vi "Interpolate 1 Table BY DP.vi"(1 "First Known Value":dbl, 7 "Psych Table, 1 Press., 1 DP":dbl[][](array[numeric])=[[1000.0, 14.17265118, 0.0, -0.621764104, 80.0, 0.000650233, 4.551631867, 12.02925562, 0.689897344, -4.171510822], [1000.0, 14.17265118, 5.0, 4.228401567, 80.0, 0.000842818, 5.899726242, 12.16386356, 2.096100991, 0.713093012], [1000.0, 14.17265118, 10.0, 9.054425448, 80.0, 0.001086491, 7.605438605, 12.29956097, 3.557591215, 5.60922632], [1000.0, 14.17265118, 15.0, 13.85608869, 80.0, 0.00139325, 9.752748458, 12.43661941, 5.08751706, 10.51277979], [1000.0, 14.17265118, 20.0, 18.63419614, 80.0, 0.001777556, 12.44289539, 12.57537024, 6.701772131, 15.41996209], [1000.0, 14.17265118, 25.0, 23.39061149, 80.0, 0.002256784, 15.79748474, 12.71621624, 8.419497627, 20.32727624], [1000.0, 14.17265118, 30.0, 28.12820033, 80.0, 0.00285173, 19.96211141, 12.85964533, 10.26367079, 25.2314979], [1000.0, 14.17265118, 35.0, 32.7497224, 80.0, 0.003529771, 24.70839817, 13.00505214, 12.19993985, 29.38106424], [1000.0, 14.17265118, 40.0, 37.4647332, 80.0, 0.004302885, 30.12019294, 13.15274062, 14.24177991, 34.32158079], [1000.0, 14.17265118, 45.0, 42.16998509, 80.0, 0.00522362, 36.56533789, 13.30388537, 16.44662842, 39.23751693], [1000.0, 14.17265118, 50.0, 46.86847898, 80.0, 0.006316212, 44.21348175, 13.45909864, 18.84172049, 44.13372432], [1000.0, 14.17265118, 55.0, 51.56310352, 80.0, 0.007608335, 53.25834337, 13.61908743, 21.45823872, 49.01435336], [1000.0, 14.17265118, 60.0, 56.25650983, 80.0, 0.009131564, 63.92094782, 13.78466719, 24.33185424, 53.88293123], [1000.0, 14.17265118, 65.0, 60.95101979, 80.0, 0.010921915, 76.45340424, 13.95677788, 27.50335816, 58.74243194], [1000.0, 14.17265118, 70.0, 65.64857135, 80.0, 0.01302048, 91.14335768, 14.13650272, 31.01940544, 63.59533911], [1000.0, 14.17265118, 75.0, 70.35069813, 80.0, 0.015474184, 108.3192857, 14.32509057, 34.93339919, 68.4437021], [1000.0, 14.17265118, 80.0, 75.05853782, 80.0, 0.018336694, 128.3568607, 14.52398268, 39.30655212, 73.28918652], [1000.0, 14.17265118, 85.0, 79.77286177, 80.0, 0.021669524, 151.6866657, 14.73484497, 44.20917244, 78.13311928], [1000.0, 14.17265118, 90.0, 84.49411846, 80.0, 0.025543377, 178.8036408, 14.9596075, 49.72223662, 82.97652911], [1000.0, 14.17265118, 95.0, 89.22248393, 80.0, 0.030039822, 210.2787556, 15.20051297, 55.93933108, 87.82018277], [1000.0, 14.17265118, 100.0, 93.95791383, 80.0, 0.035253367, 246.7735709, 15.46017708, 62.96907218, 92.66461748], [1000.0, 14.17265118, 105.0, 98.70019305, 80.0, 0.041294082, 289.0585757, 15.74166432, 70.93815137, 97.51017001], [1000.0, 14.17265118, 110.0, 103.4489805, 80.0, 0.048290929, 338.0365051, 16.04858402, 79.99520498, 102.3570026], [1000.0, 14.17265118, 115.0, 108.2038476, 80.0, 0.056396043, 394.7722978, 16.38521366, 90.31578307, 107.2051264], [1000.0, 14.17265118, 120.0, 112.9643104, 80.0, 0.065790285, 460.5319982, 16.75665854, 102.1087993, 112.0544218]], 12 "First Known Index":u16(ring) items=["DB", "WB", "RH", "HR", "Gr", "Vol", "h", "Dp"]) -> (8 "Output Array":dbl[](array[numeric]))   [LabVIEW 2020]
uses:
  <vilib>/gmath/NI_Gmath.lvlib
panel:
  out "deleted portion 1":i32
  out "Out 6":dbl
  out "Property 6":u16(ring) items=["DB", "WB", "RH", "HR", "Gr", "Vol", "h", "Dp"]
  out "deleted portion 3":i32
  out "array 3 w/ subset deleted":i32[](array[numeric])
  out "Property 5":u16(ring) items=["DB", "WB", "RH", "HR", "Gr", "Vol", "h", "Dp"]
  out "Property 4":u16(ring) items=["DB", "WB", "RH", "HR", "Gr", "Vol", "h", "Dp"]
  out "Property 3":u16(ring) items=["DB", "WB", "RH", "HR", "Gr", "Vol", "h", "Dp"]
  out "Property 2":u16(ring) items=["DB", "WB", "RH", "HR", "Gr", "Vol", "h", "Dp"]
  out "Property 1":u16(ring) items=["DB", "WB", "RH", "HR", "Gr", "Vol", "h", "Dp"]
  out "Table without elev and P":dbl[][](array[numeric])
  out "array 1 w/ subset deleted":i32[](array[numeric])
  out "Out 1":dbl
  out "Out 5":dbl
  out "Out 4":dbl
  out "Out 2":dbl
  out "Out 3":dbl
  # "will not work if DP is first known value"
  # "DB"
  # "WB"
  # "RH"
  # "HR"
  # "Gr"
  # "v"
  # "h"
  # "DP"
  # "0"
  # "1"
  # "2"
  # "3"
  # "4"
  # "5"
  # "6"
  # "7"
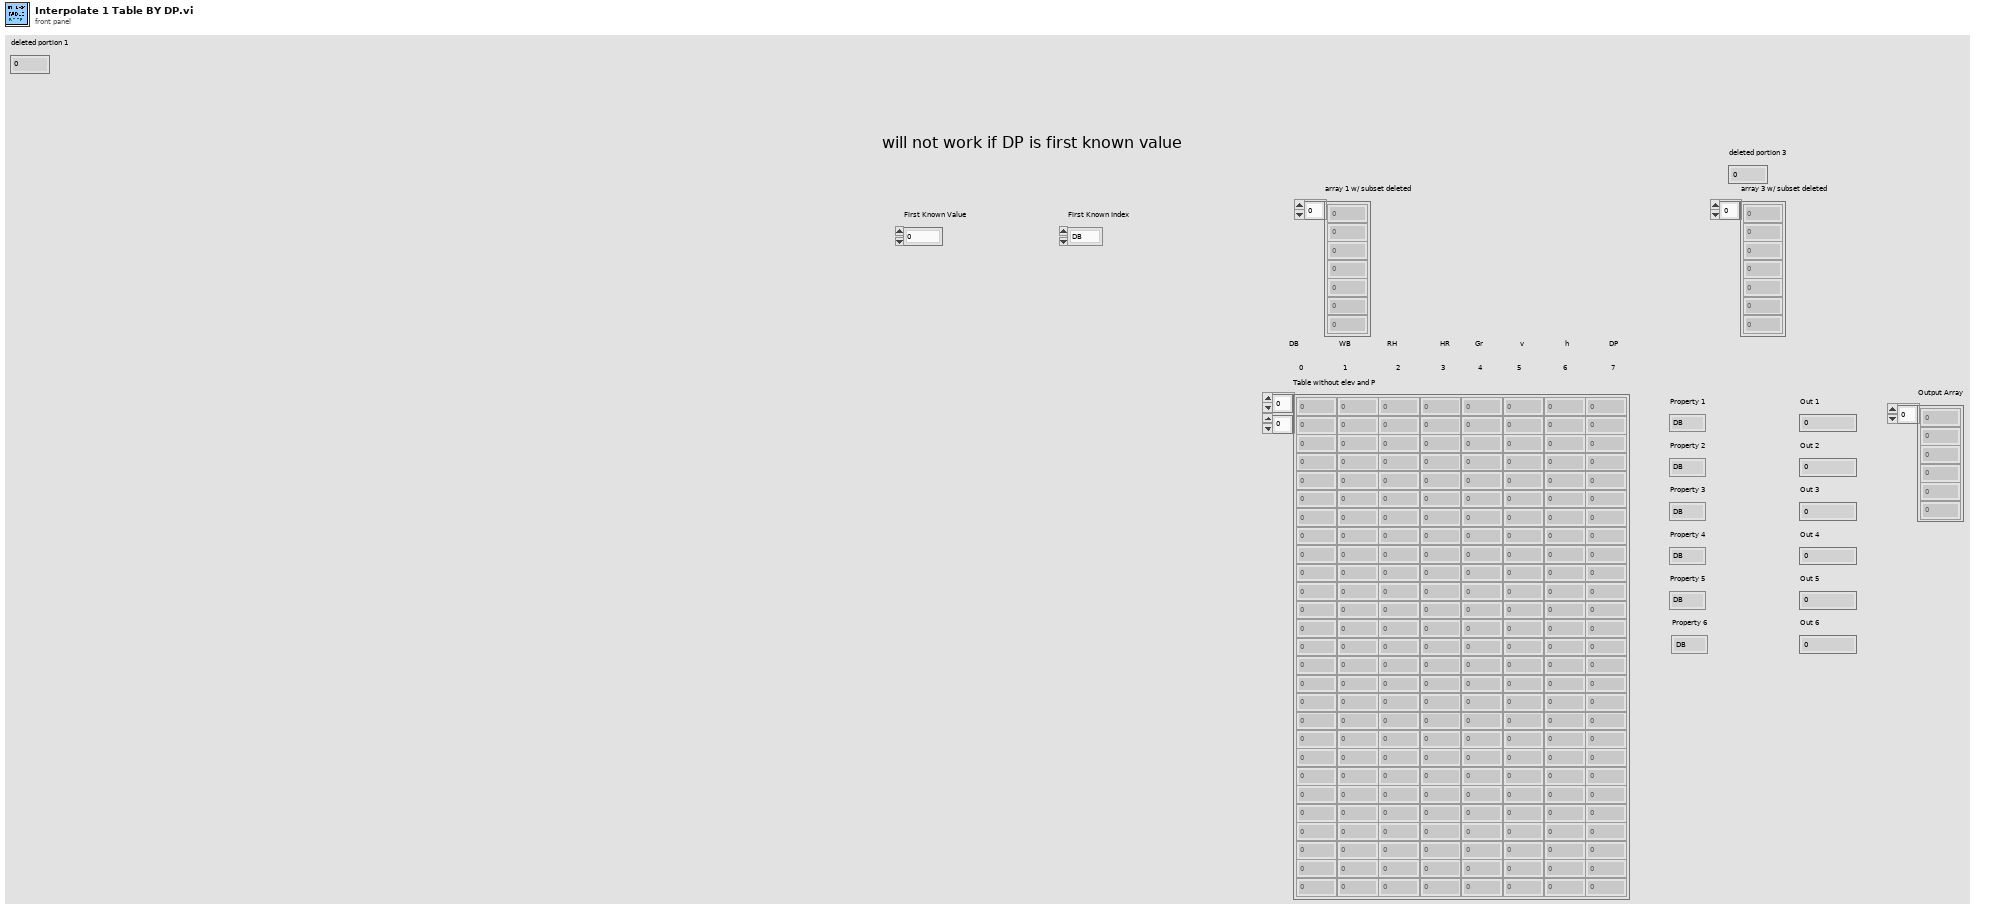
[diagram p1: front panel]
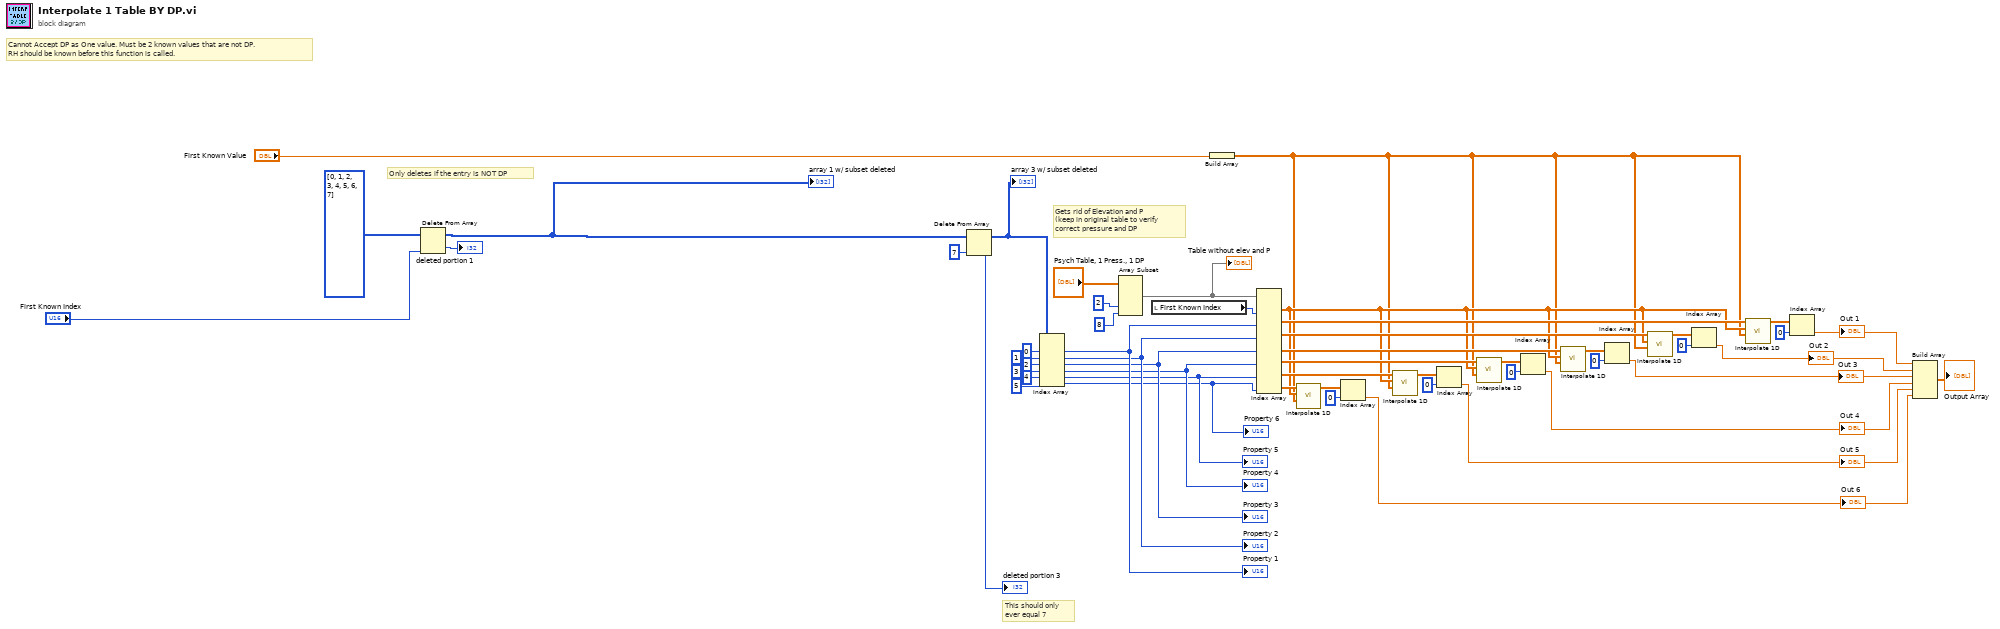
[diagram p0: block diagram]
diagram:
  # "Only deletes if the entry is NOT DP"
  # "This should only\never equal 7"
  # "Cannot Accept DP as One value. Must be 2 known values that are not DP.\nRH should be known before this function is called."
  # "Gets rid of Elevation and P \n(keep in original table to verify \ncorrect pressure and DP"
  n1 = Delete From Array(array=i32[] [0, 1, 2, 3, 4, 5, 6, 7], index="First Known Index") -> (deleted portion=→"deleted portion 1":i32, array with subset deleted=w2:i32[])  [unwired: 1 in]
  "array 1 w/ subset deleted" <- w2
  n2 = Delete From Array(array=w2, index=7) -> (deleted portion=→"deleted portion 3":i32, array with subset deleted=w22:i32[])  [unwired: 1 in]
  "array 3 w/ subset deleted" <- w22
  n3 = Index Array(array=w22, index #1=0 ("index"), index #2=1 ("index"), index #3=2 ("index"), index #4=3 ("index"), index #5=4 ("index"), index #6=5 ("index")) -> (element #1=w28:i32, element #2=w27:i32, element #3=w26:i32, element #4=w25:i32, element #5=w24:i32, element #6=w12:i32)
  "Property 1" <- w28
  "Property 2" <- w27
  "Property 3" <- w26
  "Property 4" <- w25
  "Property 5" <- w24
  "Property 6" <- w12
  n4 = Array Subset(array="Psych Table, 1 Press., 1 DP", index (col)=2 ("index"), length (col)=8 ("length")) -> (w31:dbl[][])  [unwired: 2 in]
  "Table without elev and P" <- w31
  n5 = local read "First Known Index"() -> (w20:u16)
  n6 = Build Array("First Known Value") -> (w7:dbl[])
  n7 = Index Array(array=w31, index (col) #1=w20, index (col) #2=w28, index (col) #3=w27, index (col) #4=w26, index (col) #5=w25, index (col) #6=w24, index (col) #7=w12) -> (element #1=w8:dbl[], element #2=w52:dbl[], element #3=w41:dbl[], element #4=w40:dbl[], element #5=w39:dbl[], element #6=w38:dbl[], element #7=w10:dbl[])  [unwired: 7 in]
  n8 = call <vilib>:"Interpolate 1D.vi"("xi"=w7, "X"=w8, "Y"=w10) -> ("yi"=w9:dbl[])  [unwired: 6 in, 2 out]
  n9 = Index Array(array=w9, index=0) -> (element=w6:dbl)
  "Out 6" <- w6
  n10 = call <vilib>:"Interpolate 1D.vi"("xi"=w7, "X"=w8, "Y"=w38) -> ("yi"=w43:dbl[])  [unwired: 6 in, 2 out]
  n11 = Index Array(array=w43, index=0) -> (element=w15:dbl)
  "Out 5" <- w15
  n12 = call <vilib>:"Interpolate 1D.vi"("xi"=w7, "X"=w8, "Y"=w39) -> ("yi"=w44:dbl[])  [unwired: 6 in, 2 out]
  n13 = Index Array(array=w44, index=0) -> (element=w16:dbl)
  "Out 4" <- w16
  n14 = call <vilib>:"Interpolate 1D.vi"("xi"=w7, "X"=w8, "Y"=w40) -> ("yi"=w47:dbl[])  [unwired: 6 in, 2 out]
  n15 = Index Array(array=w47, index=0) -> (element=w17:dbl)
  "Out 3" <- w17
  n16 = call <vilib>:"Interpolate 1D.vi"("xi"=w7, "X"=w8, "Y"=w41) -> ("yi"=w48:dbl[])  [unwired: 6 in, 2 out]
  n17 = Index Array(array=w48, index=0) -> (element=w18:dbl)
  "Out 2" <- w18
  n18 = call <vilib>:"Interpolate 1D.vi"("xi"=w7, "X"=w8, "Y"=w52) -> ("yi"=w51:dbl[])  [unwired: 6 in, 2 out]
  n19 = Index Array(array=w51, index=0) -> (element=w19:dbl)
  "Out 1" <- w19
  n20 = Build Array(w19, w18, w17, w16, w15, w6) -> (→"Output Array":dbl[])
